vi "Read Path.vi"(8 "error in (no error)":errorcluster, 11 "Config_Read in":refnum<class "Config_Read_BML.lvclass">) -> (0 "error out":errorcluster, 2 "Path":path, 3 "Config_Read out":refnum<class "Config_Read_BML.lvclass">)   [LabVIEW 2018, in "Config_Read_BML.lvclass"]
uses:
  Config_Read_BML.lvclass
  Config_Read_BML.lvclass/Config_Read_BML.ctl
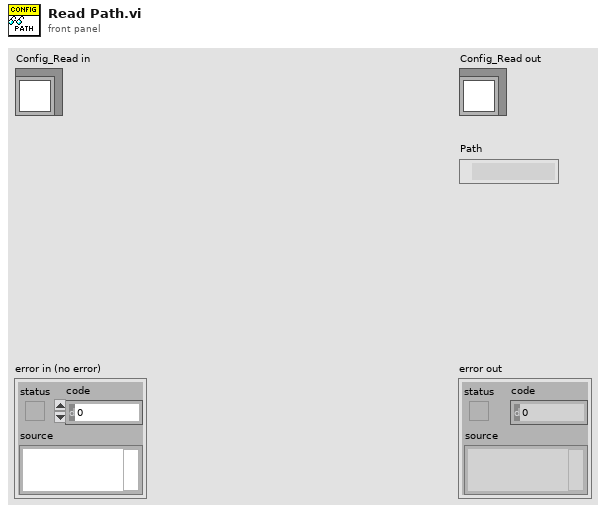
[diagram p1: front panel]
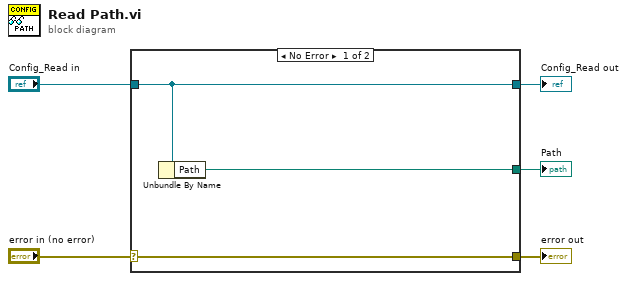
[diagram p0: block diagram]
diagram:
  n1 = case shown="No Error" "error in (no error)" {
    selector: "error in (no error)" -> [w8 w9]
    tunnel: [w8 w9] -> w4
    tunnel: [w7 w10] -> w2
    tunnel: "Config_Read in" -> [w7 w10]
    tunnel: [w6 _] -> w1
    frame No Error {
      n2 = Unbundle By Name(w7) -> ("Path"=w6:path)
    }
    frame Error {
    }
  }
  "error out" <- w4
  "Config_Read out" <- w2
  "Path" <- w1
